vi "SUGNAL GEN.vi"() -> ()   [LabVIEW 2019]
uses:
  <vilib>/Analysis/NI_AALPro.lvlib
panel:
  in  "Array":string[](array[string])
  out "Waveform Graph":dbl[](graph)
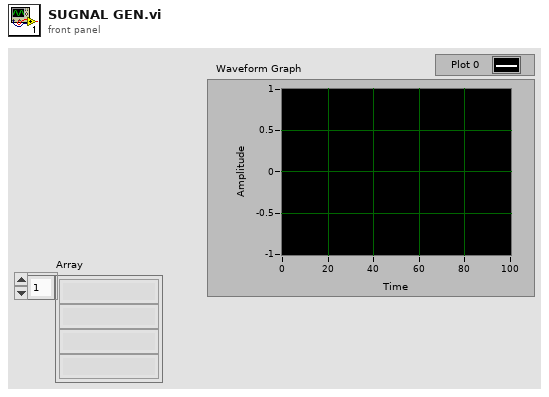
[diagram p1: front panel]
types:
  T1 = enum16{"sine", "cosine", "triangle", "square", "sawtooth", "increasing ramp", "decreasing ramp"}
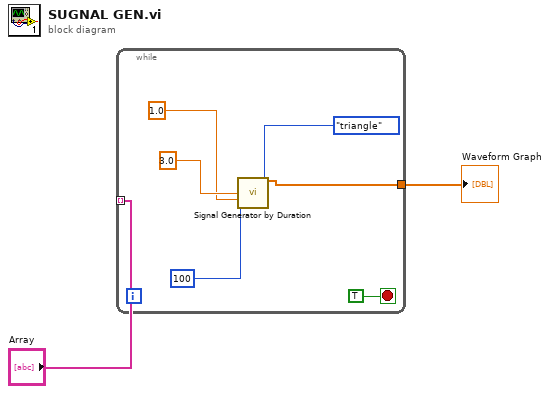
[diagram p0: block diagram]
diagram:
  n1 = while {
    tunnel: [w6] -> w2
    tunnel: "Array" -> [_] mode=indexing
    stop <- TRUE stop-if-true
    n2 = call <vilib>:"Signal Generator by Duration.vi"("signal type"=T1."triangle", "# of samples"=100, "frequency"=3.0, "amplitude"=1.0) -> ("signal"=w6:dbl[])  [unwired: 8 in, 3 out]
  }
  "Waveform Graph" <- w2
